vi "Sequencer Array.vi"() -> ()   [LabVIEW 2018]
uses:
  Test Step.ctl
  Test Result.ctl
panel:
  out "SEQUENCER Array":T1[](array[typedef]) {"Step Type" items=["Label", "Settings", "Numeric", "String", "Boolean"]}
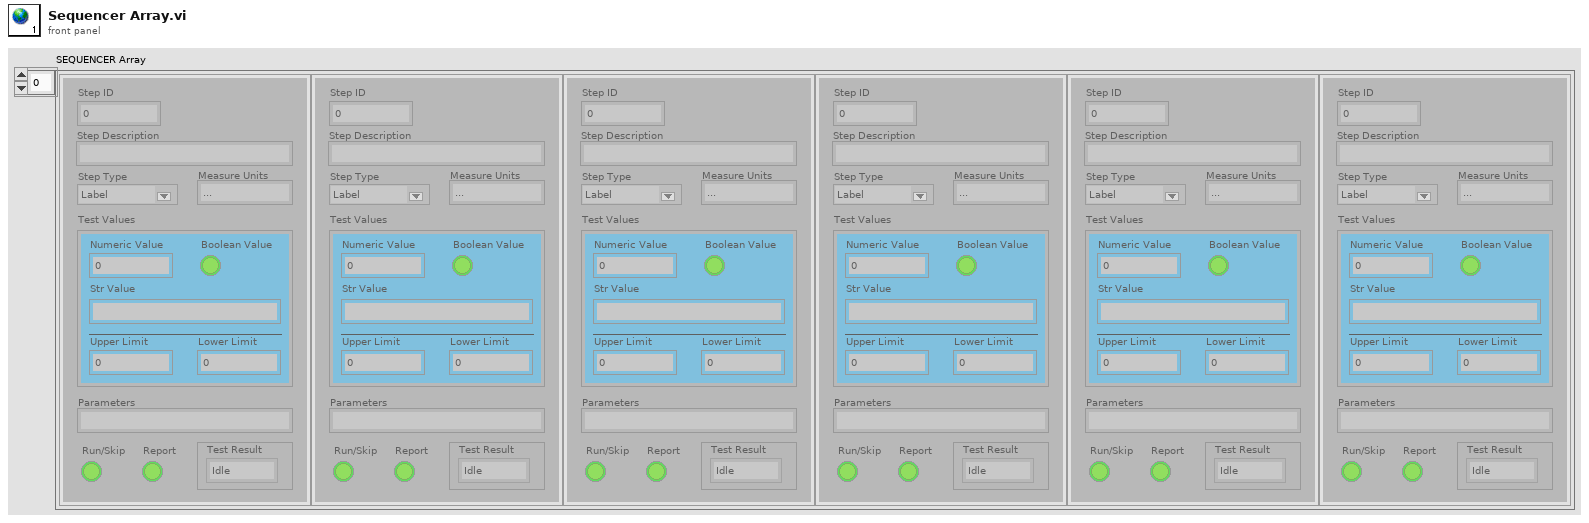
[diagram p1: front panel]
types:
  T1 = typedef "Test Step.ctl" = cluster{"Step ID":u16, "Step Description":string, "Step Type":u16, "Test Values":cluster{"Numeric Value":dbl, "Str Value":string, "Boolean Value":bool, "Upper Limit":dbl, "Lower Limit":dbl}, "Parameters":string, "Run/Skip":bool, "Test Result":T2, "Report":bool, "Measure Units":string}
  T2 = typedef "Test Result.ctl" = enum16{"Idle", "PASS", "FALSE"}
diagram:
